vi "重载控件列表.vi"(8 "error in (no error)":errorcluster caption="错误输入（无错误）", 11 "程序 输入":refnum<class "程序.lvclass">) -> (0 "error out":errorcluster caption="错误输出", 3 "程序 输出":refnum<class "程序.lvclass">)   [LabVIEW 2018, in "程序.lvclass"]
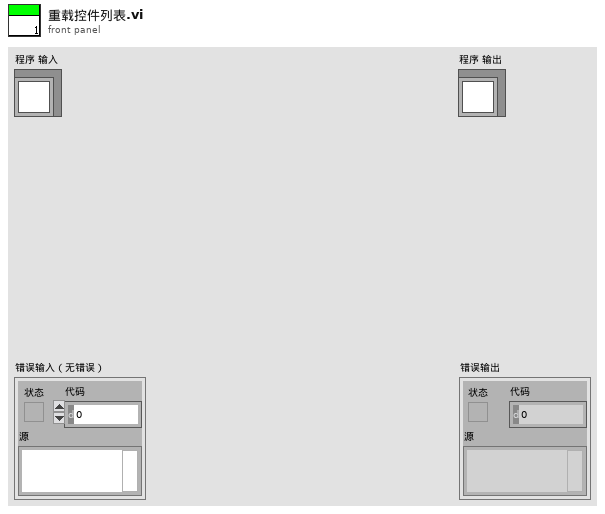
[diagram p1: front panel]
types:
  T1 = cluster{"图片":picture, "名称":string, "文本程序":string, "关键字":string}[][]
  T2 = cluster{"图片":picture, "名称":string, "文本程序":string, "关键字":string}[]
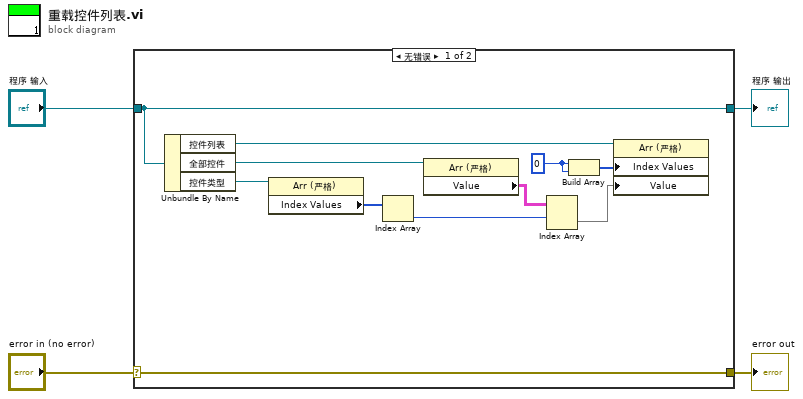
[diagram p0: block diagram]
diagram:
  n1 = case shown="无错误" "error in (no error)" {
    selector: "error in (no error)" -> [w15 w17]
    tunnel: [w15 w17] -> w3
    tunnel: [w14 w16] -> w1
    tunnel: "程序 输入" -> [w14 w16]
    frame No Error {
      w5 = u32 0
      n2 = Unbundle By Name(w14) -> ("控件列表"=w8:refnum<vi>, "全部控件"=w11:refnum<vi>, "控件类型"=w12:refnum<vi>)
      n3 = property class="Arr (严格)"(reference=w12) -> ("Index Values"=w13:u32[])  [unwired: 1 in, 2 out]
      n4 = Index Array(array=w13) -> (element=w9:u32)  [unwired: 1 in]
      n5 = property class="Arr (严格)"(reference=w11) -> ("Value"=w10:T1)  [unwired: 1 in, 2 out]
      n6 = Index Array(array=w10, index (row)=w9) -> (element=w7:T2)  [unwired: 1 in]
      n7 = Build Array(w5, w5) -> (w6:u32[])
      n8 = property class="Arr (严格)"(reference=w8, "Index Values"=w6, "Value"=w7) -> ()  [unwired: 1 in, 2 out]
    }
    frame Error {
    }
  }
  "error out" <- w3
  "程序 输出" <- w1
